vi "SetHistoryString.vi"(0 "reference in":refnum<class "Test.lvclass">, 2 "History String":string, 5 "error in (no error)":errorcluster) -> (14 "reference out":refnum<class "Test.lvclass">, 19 "error out":errorcluster)   [LabVIEW 2024, in "Test.lvclass"]
uses:
  Test.lvclass
  Test.lvclass/Test.ctl
panel:
  # "Connector Pane"
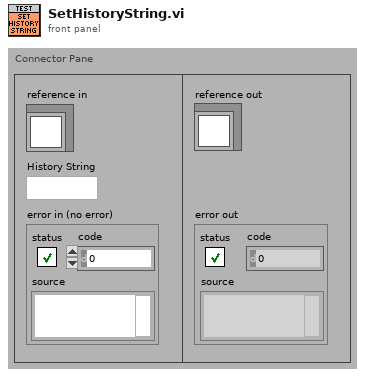
[diagram p1: front panel]
types:
  T1 = typedef "Test.lvclass/ObjectAttributes.ctl" = cluster{"Engine":bool, "Dynamometer":bool, "Test Status":enum16{"Test Start", "Test Continue", "Test Failed", "Test Success"}, "History String":string}
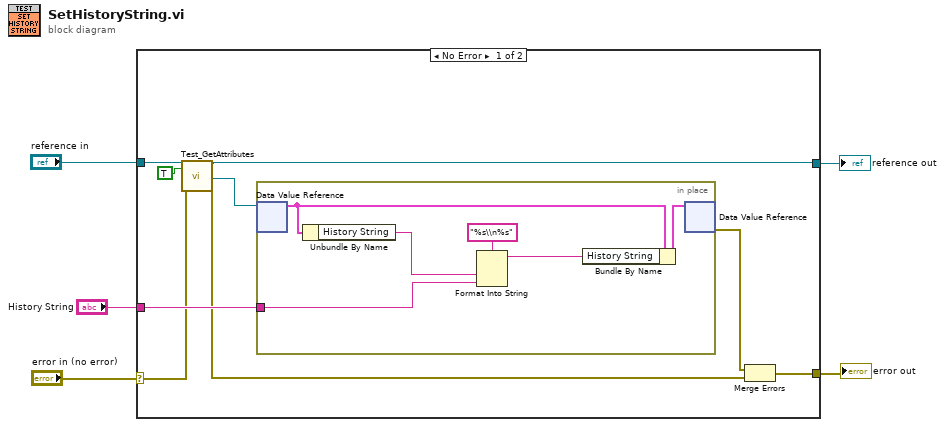
[diagram p0: block diagram]
diagram:
  n1 = case shown="No Error" "error in (no error)" {
    selector: "error in (no error)" -> [w8 w22]
    tunnel: [w12 w22] -> w4
    tunnel: [w10 w21] -> w2
    tunnel: "reference in" -> [w11 w21]
    tunnel: "History String" -> [w14 _]
    frame No Error {
      n2 = call "Test_GetAttributes.vi"("reference in"=w11, "OnlyGetDvrReference(False)"=TRUE, "error in (no error)"=w8) -> ("reference out"=w10:refnum<class "Test.lvclass">, "DataRef"=w9:refnum<data-value>, "error out"=w7:errorcluster)  [unwired: 13 in, 1 out]
      n3 = in-place {
        in-place-border: w14 -> [w16]
        n4 = in-place-dvr #1(w9) -> (w19:T1)  [unwired: 1 out]
        n5 = Unbundle By Name(w19) -> ("History String"=w17:string)
        n6 = Format Into String(format string="%s\\n%s", w17, w16) -> (resulting string=w15:string)  [unwired: 2 in, 1 out]
        n7 = Bundle By Name(cluster=w19, "History String"=w15) -> (w20:T1)
        n8 = in-place-dvr #1(w20) -> (w13:errorcluster)  [unwired: 1 out]
      }
      n9 = Merge Errors(w13, w7) -> (w12:errorcluster)
    }
    frame Error {
    }
  }
  "error out" <- w4
  "reference out" <- w2
